vi "Connection to String.vi"(11 "Connection":T1) -> (3 "String":string)   [LabVIEW 2017, in "SLSC Switch Scripting.lvlib"]
uses:
  SLSC Switch Scripting.lvlib
  Routing Channel/Connection.ctl
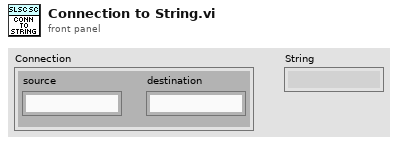
[diagram p1: front panel]
types:
  T1 = typedef "SLSC Switch Scripting.lvlib/Connection.ctl" = cluster{"source":string, "destination":string}
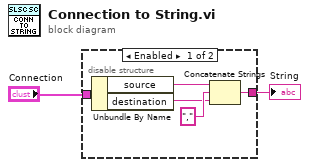
[diagram p0: block diagram]
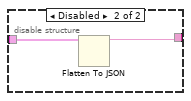
[diagram p2: hidden frame]
diagram:
  n1 = disable-structure shown="Enabled" {
    disable-tunnel: [w7 w8] -> w2
    disable-tunnel: "Connection" -> [w3 w9]
    frame Enabled {
      n2 = Unbundle By Name(w3) -> ("source"=w5:string, "destination"=w4:string)
      n3 = Concatenate Strings(w5, "," ("string"), w4) -> (w7:string)
    }
    frame Disabled {
      n4 = Flatten To JSON(anything=w9) -> (JSON string=w8:string)  [unwired: 2 in, 1 out]
    }
  }
  "String" <- w2
